vi "Angle to Stop.vi"(10 "Avg Speed":dbl format="%#_13g") -> (2 "Angle":dbl format="%#_13g")   [LabVIEW 2017]
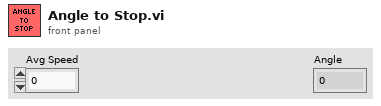
[diagram p1: front panel]
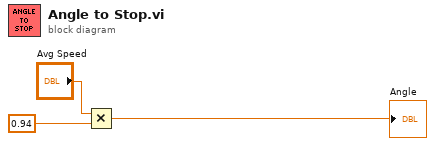
[diagram p0: block diagram]
diagram:
  n1 = Multiply(x="Avg Speed", y=0.94) -> (x*y=→"Angle":dbl)
